vi "getRecycledImagePointer.vi"(8 "error in (no error)":errorcluster, 10 "Image ID":i32, 11 "Recycled image pointer queue in":refnum<queue>) -> (0 "error out":errorcluster, 1 "Next image ID":i32, 2 "Image pointer":T1, 3 "Recycled image pointer queue out":refnum<queue>)   [LabVIEW 2017]
doc: "Either get a recycled image pointer from the queue, or create a new image pointer if there are none in the queue"
uses:
  <vilib>/vision/Image Controls.llb/IMAQ Image.ctl
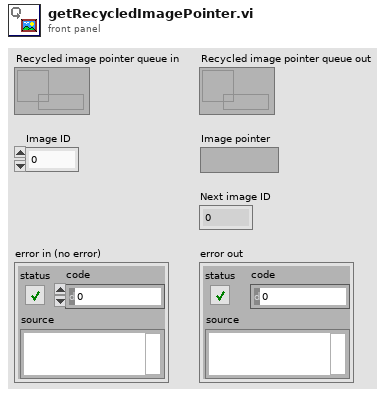
[diagram p1: front panel]
types:
  T1 = typedef "IMAQ Image.ctl" = refnum<image>
  T2 = typedef "Image Type" = u32
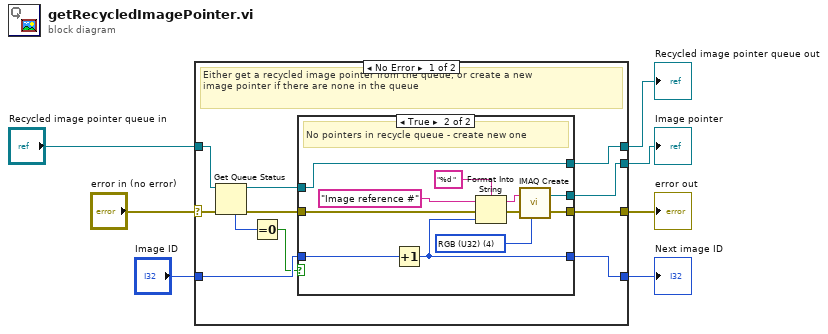
[diagram p0: block diagram]
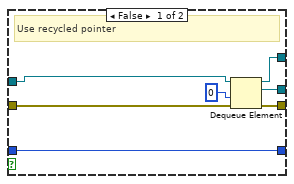
[diagram p2: hidden frame]
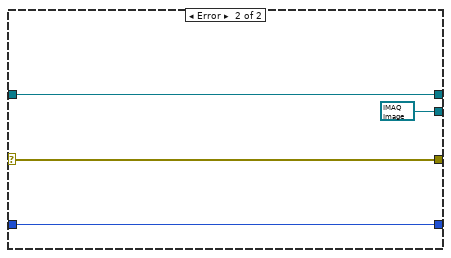
[diagram p3: hidden frame]
diagram:
  n1 = case shown="No Error" "error in (no error)" {
    selector: "error in (no error)" -> [w8 w40]
    tunnel: [w18 w40] -> w7
    tunnel: [w17 T1 refnum ("New Image")] -> w6
    tunnel: [w16 w37] -> w5
    tunnel: [w15 w39] -> w4
    tunnel: "Image ID" -> [w14 w39]
    tunnel: "Recycled image pointer queue in" -> [w11 w37]
    frame No Error {
      # "Either get a recycled image pointer from the queue, or create a new\nimage pointer if there are none in the queue"
      n2 = Get Queue Status(queue=w11, error in (no error)=w8) -> (queue out=w10:refnum<queue>, error out=w9:errorcluster, # elements in queue=w12:i32)  [unwired: 1 in, 5 out]
      n3 = Equal To 0?(x=w12) -> (x = 0?=w13:bool)
      n4 = case shown="True" w13 {
        tunnel: w14 -> [w25 w34]
        tunnel: [w25 w32] -> w15
        tunnel: w10 -> [w24 w27]
        tunnel: w9 -> [w23 w30]
        tunnel: [w21 w27] -> w16
        tunnel: [w20 w31] -> w17
        tunnel: [w19 w28] -> w18
        frame False {
          # "Use recycled pointer"
          n5 = Dequeue Element(queue=w24, timeout in ms (-1)=0, error in (no error)=w23) -> (queue out=w21:refnum<queue>, element=w20:T1, error out=w19:errorcluster)  [unwired: 1 out]
        }
        frame True {
          w26 = T2 4 items=["Grayscale (U8)", "Grayscale (I16)", "Grayscale (SGL)", "Complex (CSG)", "RGB (U32)", "HSL (U32)", "RGB (U64)", "Grayscale (U16)"] ("Image Type")
          # "No pointers in recycle queue - create new one"
          n6 = Increment(x=w34) -> (x+1=w32:i32)
          n7 = Format Into String(format string="%d " ("Image Name"), initial string="Image reference #", error in=w30, w32) -> (resulting string=w33:string, error out=w29:errorcluster)
          n8 = call "IMAQ Create"("Image Name"=w33, "Image Type"=w26, "error in (no error)"=w29) -> ("New Image"=w31:T1, "error out"=w28:errorcluster)  [unwired: 1 in, 1 out]
        }
      }
    }
    frame Error {
    }
  }
  "error out" <- w7
  "Image pointer" <- w6
  "Recycled image pointer queue out" <- w5
  "Next image ID" <- w4
